vi "Connection Notify MHLC.vi"(8 "error in (no error)":errorcluster, 10 "Data in":variant, 11 "Debug Server in":refnum<class "Debug Server.lvclass">) -> (0 "error out":errorcluster, 3 "Debug Server out":refnum<class "Debug Server.lvclass">)   [LabVIEW 2017, in "Debug Server.lvclass"]
doc: "A TCP Client connection has been established or terminated. Update Application Manager and Settings Workers correspondingly."
uses:
  Debug Server.lvclass
  C:/Program Files (x86)/National Instruments/LabVIEW 2017/vi.lib/addons/_Workers/Library/Classes/Worker/Worker.lvclass
  Settings/rqp_New Connection Log Message.ctl
  Settings/rqp_Client Connected.ctl
  Application Manager/rqp_Debug Client Disconnected.ctl
  Common VIs/DC_UID.ctl
  Debug Server.lvclass/Debug Server.ctl
  <vilib>/Utility/error.llb/Error Cluster From Error Code.vi
  <vilib>/ErrorRing/Error Ring.xnode
  Debug Server TCP Server and Client/Workers/DS TCP Server/DS TCP Server.lvclass
  Application Manager/Application Manager.lvclass
  Settings/Settings.lvclass
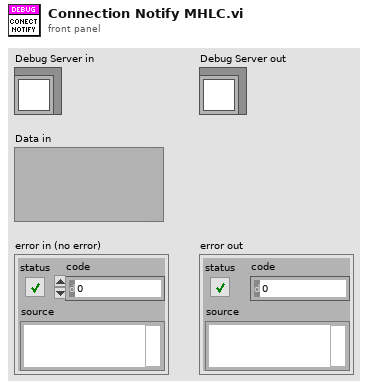
[diagram p1: front panel]
types:
  T1 = typedef "DS TCP Server.lvlib/DS TCP Server.lvclass/rsp_Connection Notify.ctl" = cluster{"Connected?":bool, "DC_UID":T2, "Message Priority":T3, "IP Address":string}
  T2 = typedef "DC_UID.ctl" = string
  T3 = typedef "Workers.lvlib/Message.lvclass/Priority.ctl" = enum16{"Low", "Normal", "High"}
  T4 = typedef "Settings.lvclass/rqp_Client Connected.ctl" = cluster{"Connected":bool}
  T5 = typedef "Settings.lvclass/rqp_New Connection Log Message.ctl" = cluster{"Message":string}
  T6 = typedef "Application Manager.lvclass/rqp_Debug Client Disconnected.ctl" = cluster{"DC_UID":T2}
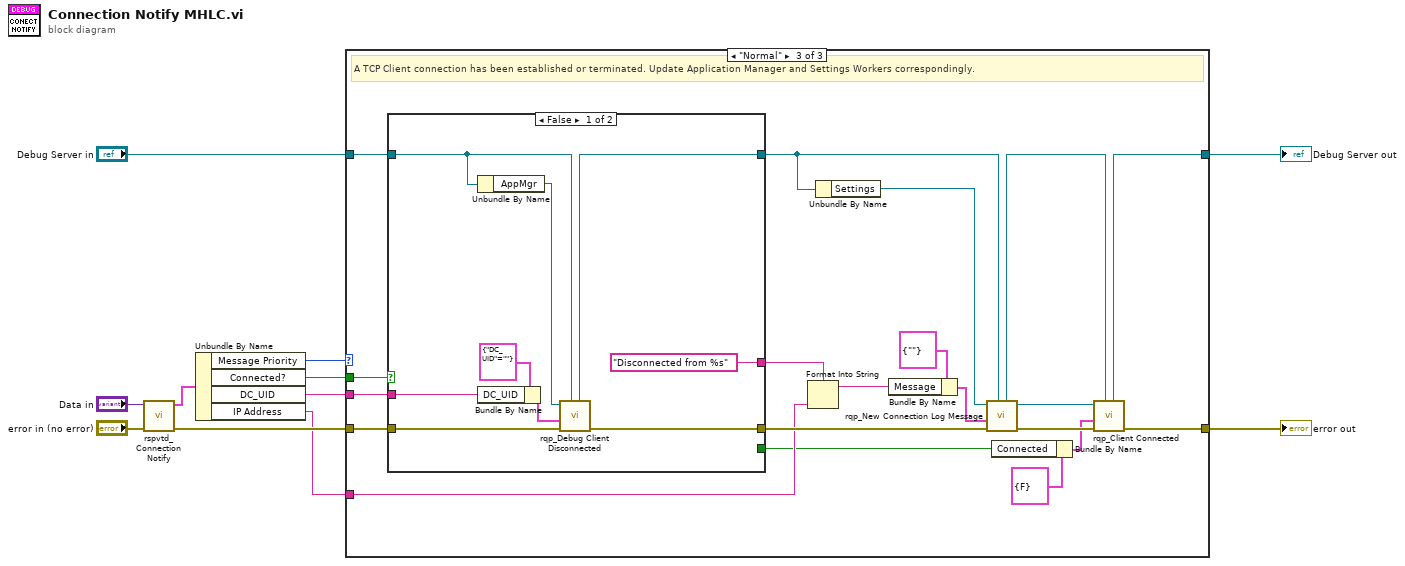
[diagram p0: block diagram]
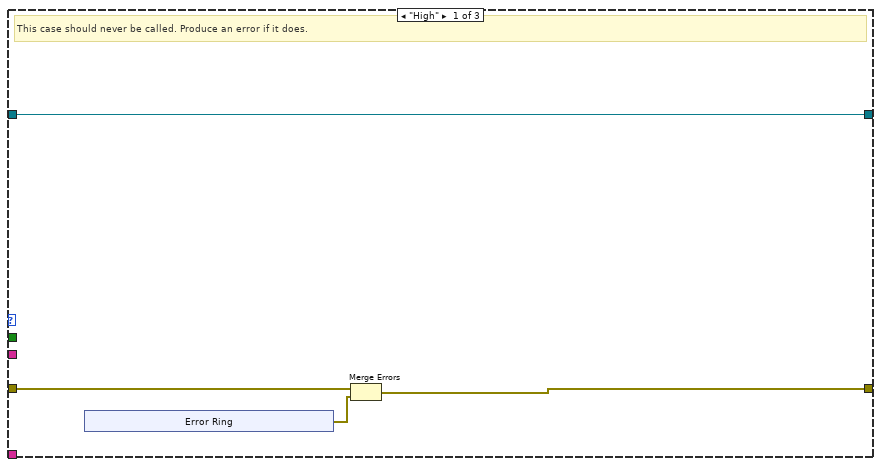
[diagram p2: hidden frame]
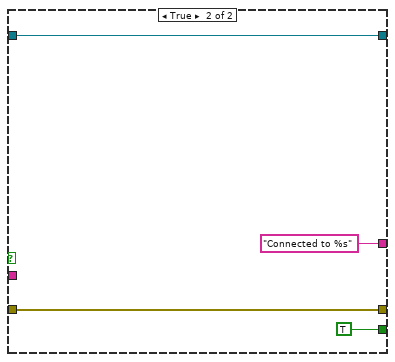
[diagram p4: hidden frame]
diagram:
  n1 = call "rspvtd_Connection Notify.vi"("error in"="error in (no error)", "Data in"="Data in") -> ("error out"=w6:errorcluster, "Data out"=w8:T1)  [unwired: 8 in]
  n2 = Unbundle By Name(w8) -> ("Message Priority"=w2:T3, "Connected?"=w4:bool, "DC_UID"=w3:T2, "IP Address"=w1:string)
  n3 = case shown="\"Normal\"" w2 {
    tunnel: "Debug Server in" -> [w15 w22 w42]
    tunnel: [w15 w22 w26] -> w10
    tunnel: [w13 w21 w29] -> w9
    tunnel: w6 -> [w14 w21 w40]
    tunnel: w4 -> [_ _ w39]
    tunnel: w3 -> [_ _ w38]
    tunnel: w1 -> [_ _ w30]
    frame "High" {
      # "This case should never be called. Produce an error if it does."
      n4 = xnode "Error Ring"() -> ("error out"=w12:errorcluster)
      n5 = Merge Errors(w14, w12) -> (w13:errorcluster)
    }
    frame "Low" {
      # "Ignore message from low prioritiy Read Workers"
    }
    frame "Normal" {
      # "A TCP Client connection has been established or terminated. Update Application Manager and Settings Workers correspondingly."
      n6 = case shown="False" w39 {
        tunnel: w42 -> [w51 w55]
        tunnel: [w50 w55] -> w36
        tunnel: [w49 w54] -> w41
        tunnel: w40 -> [w48 w54]
        tunnel: w38 -> [w47 _]
        tunnel: ["Disconnected from %s" "Connected to %s"] -> w33
        tunnel: [_ TRUE] -> w23
        frame False {
          n7 = Unbundle By Name(w51) -> ("AppMgr"=w46:refnum<class "Application Manager.lvclass">)
          n8 = Bundle By Name(cluster=T6 {"DC_UID"=""} ("Data in"), "DC_UID"=w47) -> (w44:T6)
          n9 = call "rqp_Debug Client Disconnected.vi"("Caller in"=w51, "error in"=w48, "Data in"=w44, "Application Manager in"=w46) -> ("error out"=w49:errorcluster, "dup Caller out"=w50:refnum<class "Debug Server.lvclass">)  [unwired: 5 in, 1 out]
        }
        frame True {
        }
      }
      n10 = Format Into String(format string=w33, w30) -> (resulting string=w31:string)  [unwired: 2 in, 1 out]
      n11 = Unbundle By Name(w36) -> ("Settings"=w35:refnum<class "Settings.lvclass">)
      n12 = Bundle By Name(cluster=T5 {"Message"=""} ("Data in"), "Message"=w31) -> (w32:T5)
      n13 = call "rqp_New Connection Log Message.vi"("Caller in"=w36, "error in"=w41, "Data in"=w32, "Settings in"=w35) -> ("error out"=w37:errorcluster, "dup Settings out"=w28:refnum<class "Settings.lvclass">, "dup Caller out"=w27:refnum<class "Debug Server.lvclass">)  [unwired: 5 in]
      n14 = Bundle By Name(cluster=T4 {"Connected"=FALSE} ("Data in"), "Connected"=w23) -> (w24:T4)
      n15 = call "rqp_Client Connected.vi"("Caller in"=w27, "error in"=w37, "Data in"=w24, "Settings in"=w28) -> ("error out"=w29:errorcluster, "dup Caller out"=w26:refnum<class "Debug Server.lvclass">)  [unwired: 5 in, 1 out]
    }
  }
  "Debug Server out" <- w10
  "error out" <- w9
